vi "Triggered Tasks-Stop and Clear.vi"() -> (0 "error out":errorcluster)   [LabVIEW 2017]
uses:
  Globals/gl_Triggering globals.vi
  Pockels/Globals/gl_Pockels control globals.vi
panel:
  in  "error in":errorcluster
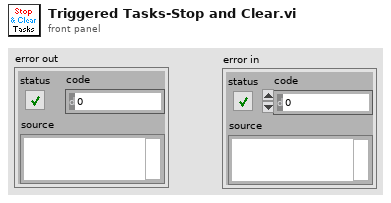
[diagram p1: front panel]
types:
  T1 = typedef "Triggered tasks cluster.ctl" = cluster{"DO task-Encoder trigger":refnum<k21>, "AO Task-Pockels modulation":refnum<k21>, "Counter Clock Task":refnum<k21>}
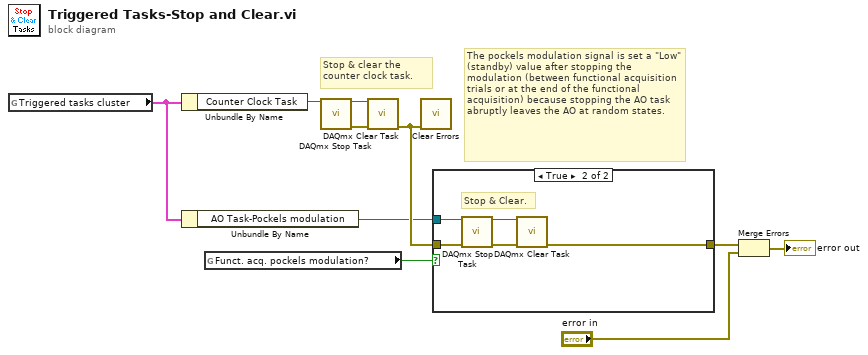
[diagram p0: block diagram]
diagram:
  # "The pockels modulation signal is set a \"Low\" (standby) value after stopping the modulation (between functional acquisition trials or at the end of the functional acquisition) because stopping the AO task abruptly leaves the AO at random states."
  # "Stop & clear the counter clock task."
  n1 = global read "gl_Triggering globals.vi" "Triggered tasks cluster"() -> (w5:T1)
  n2 = Unbundle By Name(w5) -> ("Counter Clock Task"=w8:refnum<k21>)
  n3 = Unbundle By Name(w5) -> ("AO Task-Pockels modulation"=w6:refnum<k21>)
  n4 = global read "gl_Pockels control globals.vi" "Funct. acq. pockels modulation?"() -> (w7:bool)
  n5 = call <vilib>:"DAQmx Stop Task.vi"("task/channels in"=w8) -> ("task out"=w4:refnum<k21>, "error out"=w3:errorcluster)  [unwired: 13 in]
  n6 = call <vilib>:"DAQmx Clear Task.vi"("task in"=w4, "error in"=w3) -> ("error out"=w10:errorcluster)  [unwired: 13 in]
  n7 = call <vilib>:"Clear Errors.vi"("error in (no error)"=w10) -> ()  [unwired: 5 in, 2 out]
  n8 = case shown="True" w7 {
    tunnel: [w11 w12] -> w9
    tunnel: w6 -> [_ w14]
    tunnel: w10 -> [w11 w13]
    frame False {
    }
    frame True {
      # "Stop & Clear."
      n9 = call <vilib>:"DAQmx Stop Task.vi"("task/channels in"=w14, "error in"=w13) -> ("task out"=w16:refnum<k21>, "error out"=w15:errorcluster)  [unwired: 12 in]
      n10 = call <vilib>:"DAQmx Clear Task.vi"("task in"=w16, "error in"=w15) -> ("error out"=w12:errorcluster)  [unwired: 13 in]
    }
  }
  n11 = Merge Errors(w9, "error in") -> (→"error out":errorcluster)
